vi "Set A delay.vi"(8 "error in (no error)":errorcluster, 10 "A delay":string, 11 "Sync Box in":refnum<class "Sync Box.lvclass">) -> (0 "error out":errorcluster, 3 "Sync Box out":refnum<class "Sync Box.lvclass">)   [LabVIEW 2018, in "Sync Box.lvclass"]
uses:
  Sync Box.lvclass
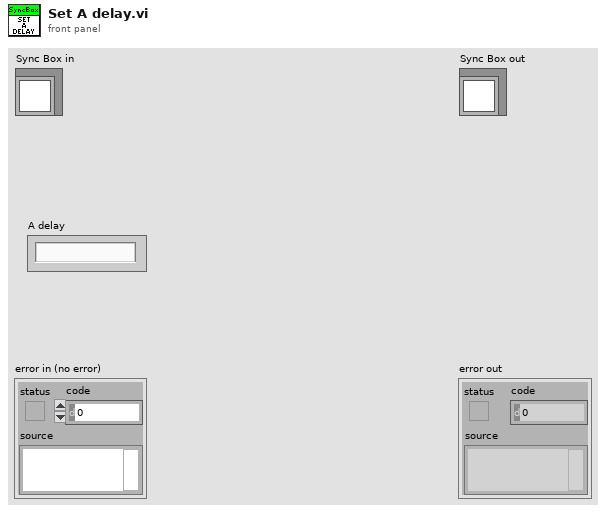
[diagram p1: front panel]
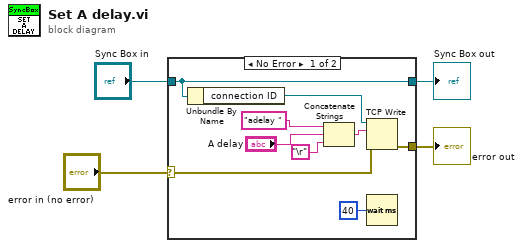
[diagram p0: block diagram]
diagram:
  n1 = case shown="No Error" "error in (no error)" {
    selector: "error in (no error)" -> [w9 w15]
    tunnel: [w8 w15] -> w3
    tunnel: [w10 w14] -> w1
    tunnel: "Sync Box in" -> [w10 w14]
    frame No Error {
      n2 = Unbundle By Name(w10) -> ("connection ID"=w13:refnum<k5>)
      n3 = Concatenate Strings("adelay ", "A delay", "\r") -> (w12:string)
      n4 = TCP Write(connection ID=w13, data in=w12, error in (no error)=w9) -> (error out=w8:errorcluster)  [unwired: 1 in, 2 out]
      n5 = Wait (ms)(milliseconds to wait=u32 40) -> ()  [unwired: 1 out]
    }
    frame Error {
    }
  }
  "error out" <- w3
  "Sync Box out" <- w1
